vi "Stop Core.vi"(10 "final error code":i32, 11 "BuildWorker in":refnum<class "BuildWorker.lvclass">) -> (3 "BuildWorker out":refnum<class "BuildWorker.lvclass">)   [LabVIEW 2017, in "BuildWorker.lvlib" / "BuildWorker.lvclass"]
doc: "(<B>Filename</B>: Actor Framework.lvlib:Actor.lvclass:Stop Core.vi)\n\nDefines what the actor does before it stops. Use the <B>final error code</B> input to determine whether the actor shut down in response to an error.\n\nBy default, this method does nothing. A descendant class may override it to define behavior, such as shutting down any processes the actor initiated in its override of the Actor Core method."
uses:
  BuildWorker.lvclass
  BuildWorker.lvclass/BuildWorker.ctl
  WebSocket Server/Actors/Actor wHelper/Actor wUI/Actor wUI.lvclass
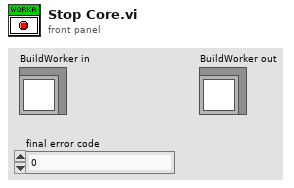
[diagram p1: front panel]
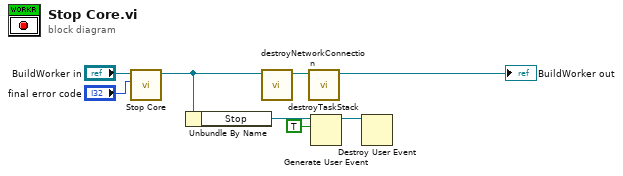
[diagram p0: block diagram]
diagram:
  n1 = call-parent "Stop Core.vi"("final error code"="final error code", "Actor wUI in"="BuildWorker in") -> ("Actor wUI out"=w6:refnum<class "BuildWorker.lvclass">)  [unwired: 9 in]
  n2 = Unbundle By Name(w6) -> ("Stop"=w5:refnum<user-event>)
  n3 = call "destroyNetworkConnection.vi"("BuildWorker in"=w6) -> ("BuildWorker out"=w2:refnum<class "BuildWorker.lvclass">)  [unwired: 9 in, 1 out]
  n4 = call "destroyTaskStack.vi"("BuildWorker in"=w2) -> ("BuildWorker out"=→"BuildWorker out":refnum<class "BuildWorker.lvclass">)  [unwired: 9 in, 1 out]
  n5 = Generate User Event(user event=w5, event data cluster=TRUE ("event data")) -> (user event out=w4:refnum<user-event>)  [unwired: 2 in, 1 out]
  n6 = Destroy User Event(user event=w4) -> ()  [unwired: 1 in, 1 out]
